vi "Shorten Class name.vi"(1 "Name.lvclass":string) -> (0 "Name":string)   [LabVIEW 2019, in "Control Experiment.lvclass"]
uses:
  Control Experiment.lvclass
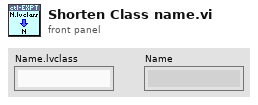
[diagram p1: front panel]
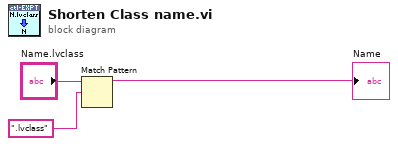
[diagram p0: block diagram]
diagram:
  n1 = Match Pattern(string="Name.lvclass", regular expression=".lvclass") -> (before substring=→"Name":string)  [unwired: 1 in, 3 out]
